vi "Control Loop Process.vi"(8 "error in (no error)":errorcluster, 9 "MainDirectionIn":string, 11 "Main Process Class in":refnum<class "MPC_VirbVision.lvclass">) -> (0 "error out":errorcluster, 1 "MainDirectionOut":string, 2 "ProcessAction":string[](array[string]), 3 "Main Process Class out":refnum<class "MPC_VirbVision.lvclass">)   [LabVIEW 2019, in "MPC_VirbVision.lvclass"]
uses:
  MPC_VirbVision.lvclass
  Main Class.lvclass
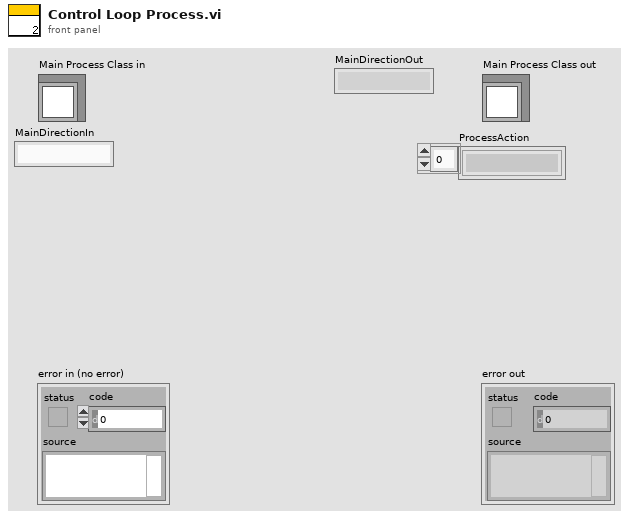
[diagram p1: front panel]
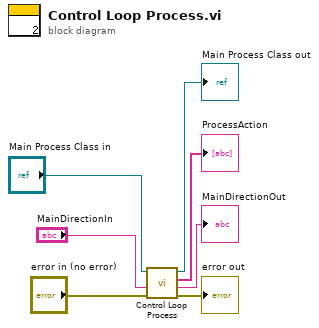
[diagram p0: block diagram]
diagram:
  n1 = call-parent "Control Loop Process.vi"("error in (no error)"="error in (no error)", "MainDirectionIn"="MainDirectionIn", "Main Process Class in"="Main Process Class in") -> ("error out"=→"error out":errorcluster, "MainDirectionOut"=→"MainDirectionOut":string, "ProcessAction"=→"ProcessAction":string[], "Main Process Class out"=→"Main Process Class out":refnum<class "MPC_VirbVision.lvclass">)  [unwired: 5 in]
